vi "FTW-App-StringToVersion.vi"(0 "Version String":string) -> (1 "Major":i32, 2 "Minor":i32, 3 "Fix":i32, 4 "Build":i32)   [LabVIEW 2015]
panel:
  # "Inputs"
  # "Outputs"
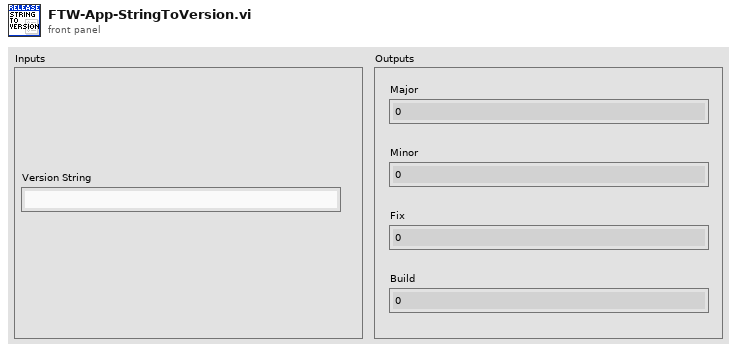
[diagram p1: front panel]
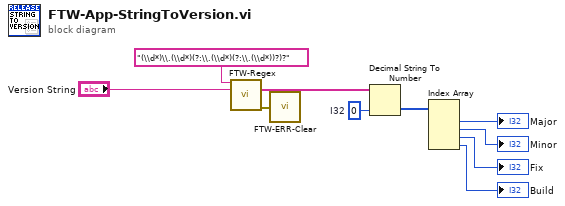
[diagram p0: block diagram]
diagram:
  w6 = 0  # I32
  n1 = call "FTW-Regex.vi"("Regular Expression"="(\\d*)\\.(\\d*)(?:\\.(\\d*)(?:\\.(\\d*))?)?" ("regular expression"), "Input String"="Version String") -> ("Submatches"=w2:string[], "error out"=w1:errorcluster)  [unwired: 9 in, 3 out]
  n2 = call "FTW-ERR-Clear.vi"("error to snuff"=w1) -> ()  [unwired: 1 out]
  n3 = Decimal String To Number(string=w2, default (0L)=w6) -> (number=w5:i32[])  [unwired: 1 in, 1 out]
  n4 = Index Array(array=w5) -> (element #1=→"Major":i32, element #2=→"Minor":i32, element #3=→"Fix":i32, element #4=→"Build":i32)  [unwired: 4 in]
